vi "Is Cell In Table.vi"(0 "Cell":cluster{"Row":i32, "Column":i32}, 7 "Size":cluster{"Rows":i32, "Columns":i32}) -> (4 "Cell thru":cluster{"Row":i32, "Column":i32}, 8 "in table":bool)   [LabVIEW 2020, in "KTable.xctl"]
uses:
  KTable.xctl
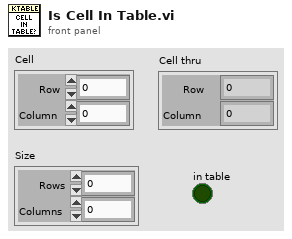
[diagram p1: front panel]
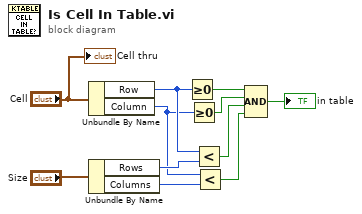
[diagram p0: block diagram]
diagram:
  n1 = Unbundle By Name("Cell") -> ("Row"=w5:i32, "Column"=w3:i32)
  n2 = Unbundle By Name("Size") -> ("Rows"=w9:i32, "Columns"=w8:i32)
  n3 = Greater Or Equal To 0?(x=w5) -> (x >= 0?=w4:bool)
  n4 = Greater Or Equal To 0?(x=w3) -> (x >= 0?=w2:bool)
  n5 = Less?(x=w5, y=w9) -> (x < y?=w7:bool)
  n6 = Less?(x=w3, y=w8) -> (x < y?=w6:bool)
  n7 = Compound Arithmetic op=AND(w4, w2, w7, w6) -> (→"in table":bool)
  "Cell thru" <- "Cell"
